vi "scaling matrix.vi"(5 "universal y-scale":dbl, 7 "Scale":u16(ring) items=["no scaling", "universal scaling", "1st row", "matrix", "frequency (matrix)", "freq. 1st col. (real 1, im 1, re 2, im 2, ....)"], 9 "row index":i32, 10 "col index":i32, 11 "scale matrix":dbl[][](array[numeric])=[[1000.0, -1000.0, 200000.0, 1.0, 1.0, 1.0], [2000.0, -500.0, 1000000.0, 0.0, 0.0, 0.0], [5000.0, -1000.0, 1000000.0, 0.0, 0.0, 0.0], [10000.0, -2000.0, 1000000.0, 0.0, 0.0, 0.0], [20000.0, -5000.0, 1000000.0, 0.0, 0.0, 0.0], [500.0, -1000.0, 0.0, 0.0, 0.0, 0.0], [500.0, -40000.0, 0.0, 0.0, 0.0, 0.0], [500.0, -45000.0, 0.0, 0.0, 0.0, 0.0], [500.0, -50000.0, 0.0, 0.0, 0.0, 0.0], [500.0, -1000.0, 0.0, 0.0, 0.0, 0.0], [2000.0, -2000.0, 0.0, 0.0, 0.0, 0.0], [2000.0, -2000.0, 0.0, 0.0, 0.0, 0.0], [4000.0, -4000.0, 0.0, 0.0, 0.0, 0.0], [4000.0, -4000.0, 0.0, 0.0, 0.0, 0.0]] format="%#_6e") -> (3 "scale\nfactor":dbl)   [LabVIEW 2021]
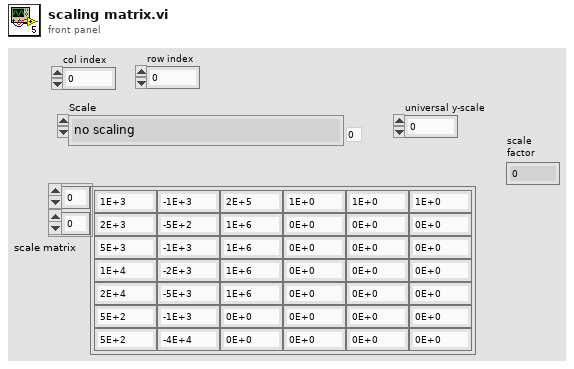
[diagram p1: front panel]
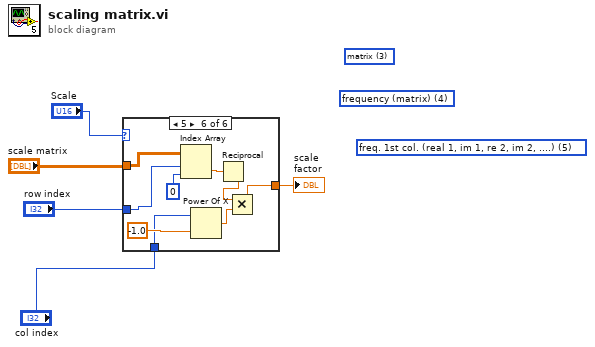
[diagram p0: block diagram]
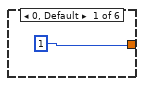
[diagram p2: hidden frame]
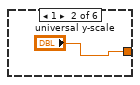
[diagram p3: hidden frame]
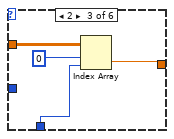
[diagram p4: hidden frame]
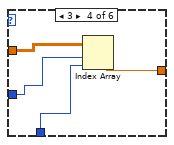
[diagram p5: hidden frame]
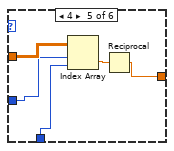
[diagram p6: hidden frame]
diagram:
  (unwired) u16 5 items=["no scaling", "universal scaling", "1st row", "matrix", "frequency (matrix)", "freq. 1st col. (real 1, im 1, re 2, im 2, ....)"] ("Scale")
  (unwired) u16 4 items=["no scaling", "universal scaling", "1st row", "matrix", "frequency (matrix)", "freq. 1st col. (real 1, im 1, re 2, im 2, ....)"] ("Scale")
  (unwired) u16 3 items=["no scaling", "universal scaling", "1st row", "matrix", "frequency (matrix)", "freq. 1st col. (real 1, im 1, re 2, im 2, ....)"] ("Scale")
  n1 = case shown="5" "Scale" {
    tunnel: [1 "universal y-scale" w9 w14 w18 w23] -> w1
    tunnel: "row index" -> [_ _ _ w13 w17 w22]
    tunnel: "scale matrix" -> [_ _ w11 w15 w20 w29]
    tunnel: "col index" -> [_ _ w8 w12 w16 w21]
    frame 0, Default {
    }
    frame 1 {
    }
    frame 2 {
      n2 = Index Array(array=w11, index (row)=0, index (col)=w8) -> (element=w9:dbl)
    }
    frame 3 {
      n3 = Index Array(array=w15, index (row)=w13, index (col)=w12) -> (element=w14:dbl)
    }
    frame 4 {
      n4 = Index Array(array=w20, index (row)=w17, index (col)=w16) -> (element=w19:dbl)
      n5 = Reciprocal(x=w19) -> (1/x=w18:dbl)
    }
    frame 5 {
      n6 = Index Array(array=w29, index (row)=w22, index (col)=0 ("disabled index (col)")) -> (element=w28:dbl)
      n7 = Power Of X(1:-1.0 ("x"), 2:w21) -> (0:w25:dbl)
      n8 = Reciprocal(x=w28) -> (1/x=w24:dbl)
      n9 = Multiply(x=w24, y=w25) -> (x*y=w23:dbl)
    }
  }
  "scale\nfactor" <- w1
